vi "Control_Turbi_BIn.vi"(0 "Manual_Off":T1, 1 "Estados_IN":bool[](array[boolean]), 7 "Error In":errorcluster, 8 "T-On (s)":dbl) -> (20 "Estados_OUT":bool[](array[boolean]), 27 "Error Out":errorcluster)   [LabVIEW 2013]
uses:
  Controles/Manual_OFF_TB.ctl
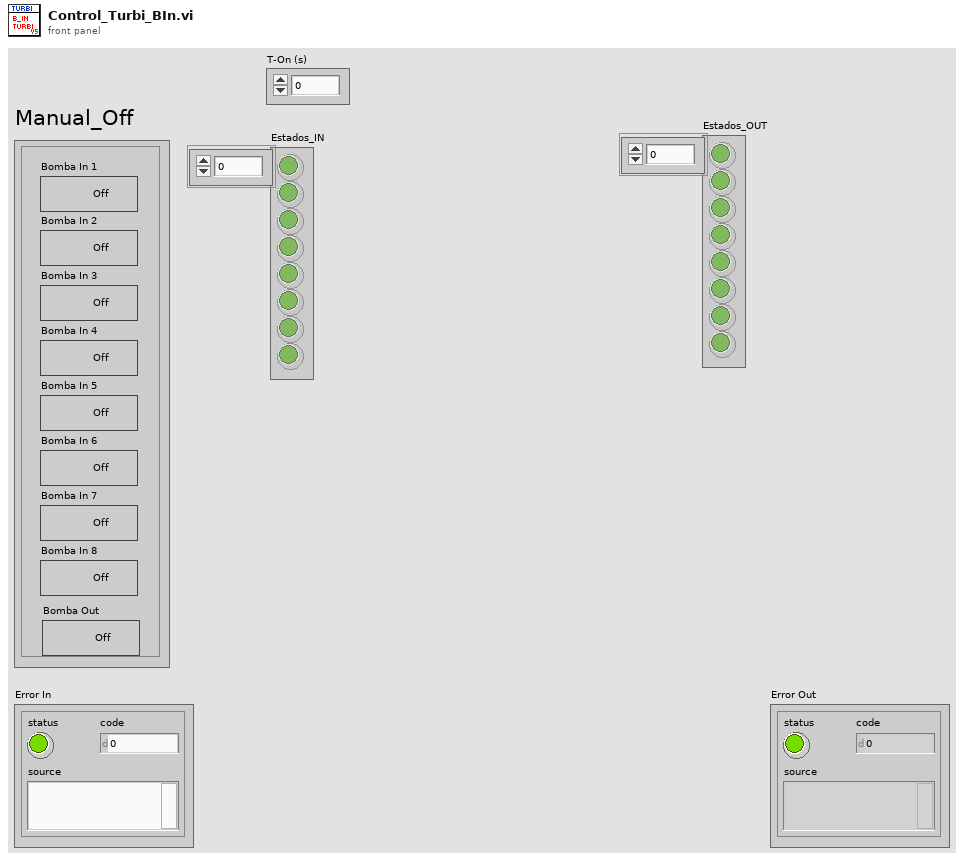
[diagram p1: front panel]
types:
  T1 = typedef "Manual_OFF_TB.ctl" = cluster{"Bomba In 1-1":bool, "Bomba In 1-2":bool, "Bomba In 1-3":bool, "Bomba In 1-4":bool, "Bomba In 1-5":bool, "Bomba In 1-6":bool, "Bomba In 1-7":bool, "Bomba In 1-8":bool, "Bomba Out1":bool}
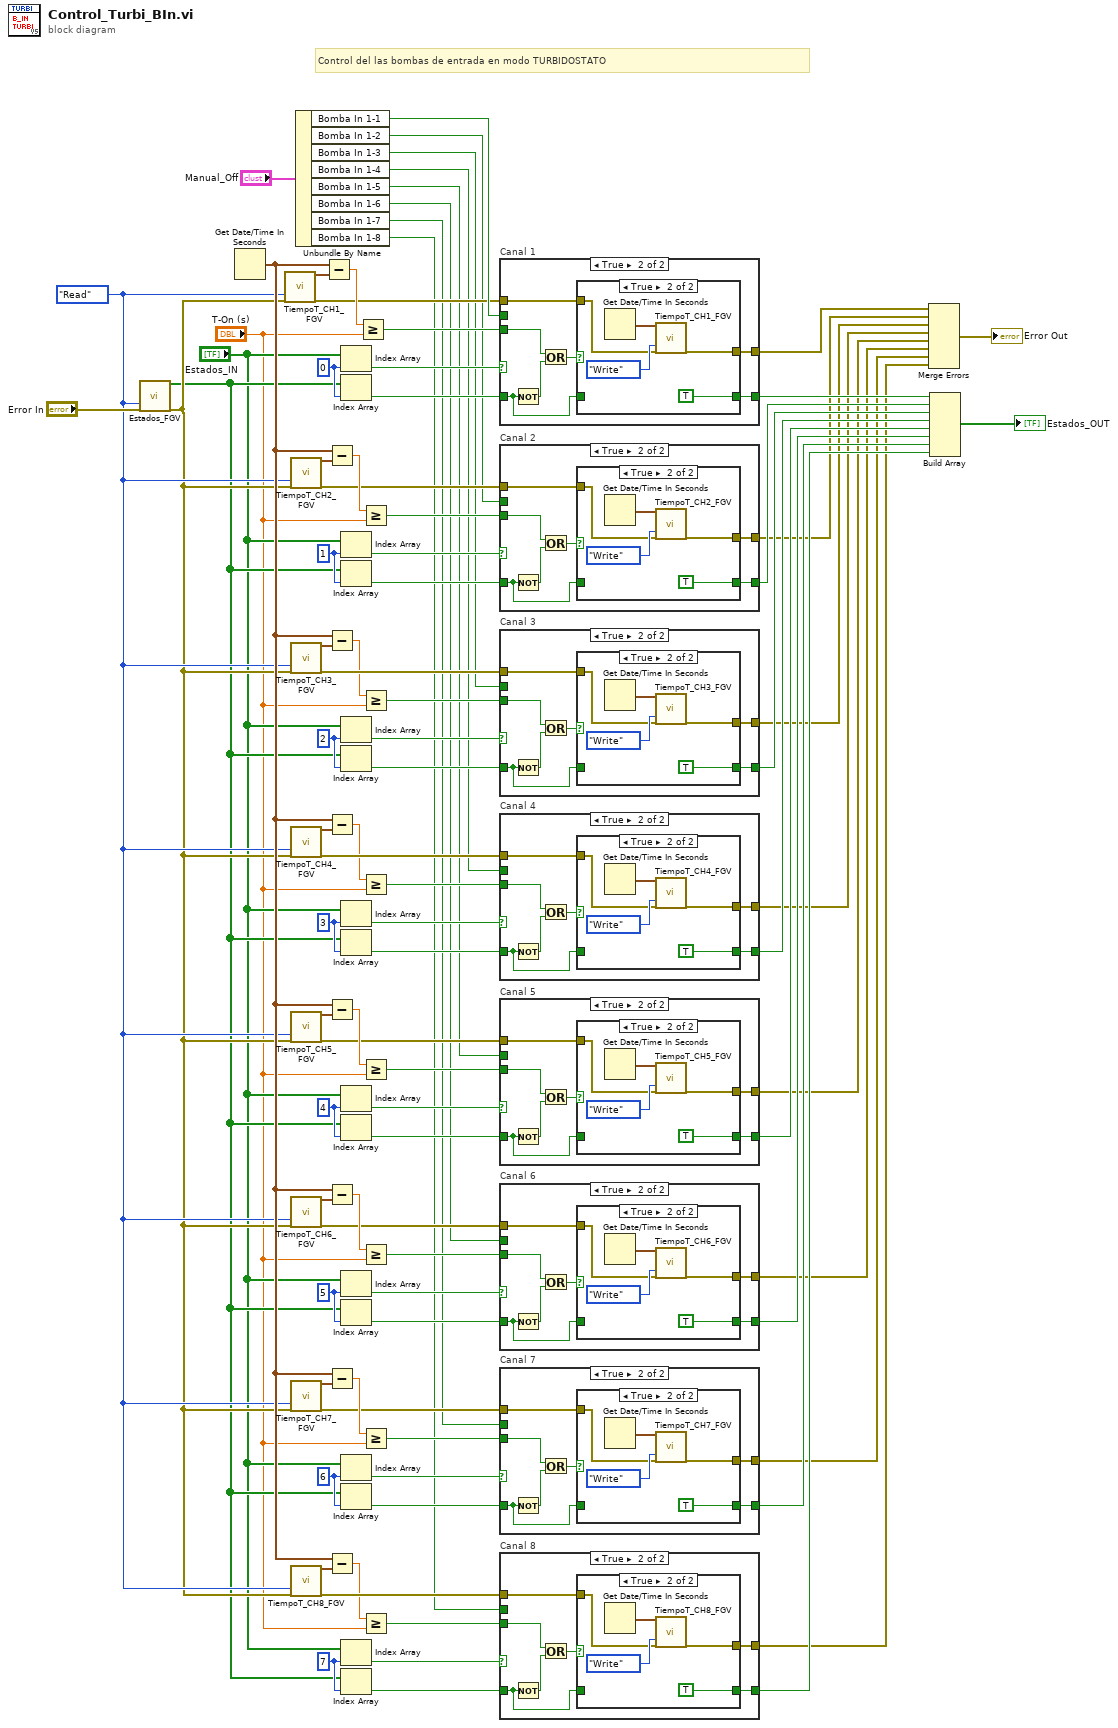
[diagram p0: block diagram]
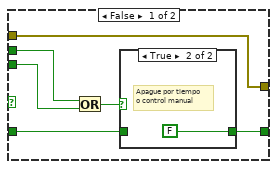
[diagram p2: hidden frame]
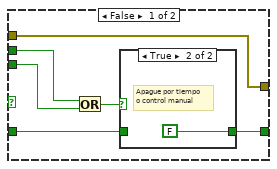
[diagram p5: hidden frame]
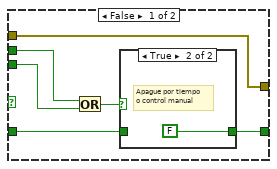
[diagram p8: hidden frame]
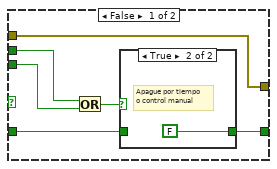
[diagram p11: hidden frame]
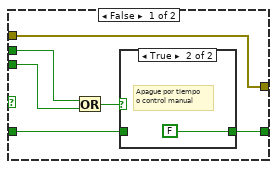
[diagram p14: hidden frame]
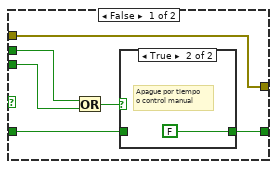
[diagram p17: hidden frame]
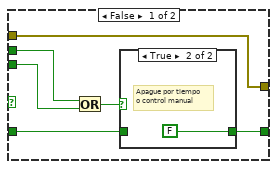
[diagram p20: hidden frame]
diagram:
  w30 = 7 ("index")
  w41 = 6 ("index")
  w27 = 5 ("index")
  w59 = 4 ("index")
  w48 = 3 ("index")
  w64 = 2 ("index")
  w77 = 1 ("index")
  w17 = enum16{"Write", "Read"}."Read" ("Opción")
  w82 = 0 ("index")
  # "Control del las bombas de entrada en modo TURBIDOSTATO"
  n1 = call "Estados_FGV.vi"("Opción"=w17, "Error In"="Error In") -> ("Estados_OUT"=w15:bool[], "Error Out"=w16:errorcluster)  [unwired: 16 in]
  n2 = Get Date/Time In Seconds() -> (seconds since 1Jan1904=w18:timestamp)
  n3 = call "TiempoT_CH1_FGV.vi"("Opción"=w17, "Error In"=w16) -> ("Tiempo_OUT"=w89:timestamp, "Error Out"=w84:errorcluster)  [unwired: 15 in, 1 out]
  n4 = call "TiempoT_CH2_FGV.vi"("Opción"=w17, "Error In"=w16) -> ("Tiempo_OUT"=w72:timestamp, "Error Out"=w73:errorcluster)  [unwired: 15 in, 1 out]
  n5 = call "TiempoT_CH3_FGV.vi"("Opción"=w17, "Error In"=w16) -> ("Tiempo_OUT"=w69:timestamp, "Error Out"=w68:errorcluster)  [unwired: 15 in, 1 out]
  n6 = call "TiempoT_CH4_FGV.vi"("Opción"=w17, "Error In"=w16) -> ("Tiempo_OUT"=w53:timestamp, "Error Out"=w52:errorcluster)  [unwired: 15 in, 1 out]
  n7 = call "TiempoT_CH5_FGV.vi"("Opción"=w17, "Error In"=w16) -> ("Tiempo_OUT"=w54:timestamp, "Error Out"=w55:errorcluster)  [unwired: 15 in, 1 out]
  n8 = call "TiempoT_CH6_FGV.vi"("Opción"=w17, "Error In"=w16) -> ("Tiempo_OUT"=w22:timestamp, "Error Out"=w23:errorcluster)  [unwired: 15 in, 1 out]
  n9 = call "TiempoT_CH7_FGV.vi"("Opción"=w17, "Error In"=w16) -> ("Tiempo_OUT"=w36:timestamp, "Error Out"=w37:errorcluster)  [unwired: 15 in, 1 out]
  n10 = call "TiempoT_CH8_FGV.vi"("Opción"=w17, "Error In"=w16) -> ("Tiempo_OUT"=w35:timestamp, "Error Out"=w34:errorcluster)  [unwired: 15 in, 1 out]
  n11 = Unbundle By Name("Manual_Off") -> ("Bomba In 1-1"=w85:bool, "Bomba In 1-2"=w70:bool, "Bomba In 1-3"=w61:bool, "Bomba In 1-4"=w44:bool, "Bomba In 1-5"=w43:bool, "Bomba In 1-6"=w12:bool, "Bomba In 1-7"=w11:bool, "Bomba In 1-8"=w10:bool)
  n12 = Subtract(x=w18, y=w89) -> (x-y=w88:dbl)
  n13 = Subtract(x=w18, y=w72) -> (x-y=w75:dbl)
  n14 = Subtract(x=w18, y=w69) -> (x-y=w66:dbl)
  n15 = Subtract(x=w18, y=w53) -> (x-y=w50:dbl)
  n16 = Subtract(x=w18, y=w54) -> (x-y=w57:dbl)
  n17 = Subtract(x=w18, y=w22) -> (x-y=w25:dbl)
  n18 = Subtract(x=w18, y=w36) -> (x-y=w39:dbl)
  n19 = Subtract(x=w18, y=w35) -> (x-y=w32:dbl)
  n20 = Index Array(array="Estados_IN", index=w82) -> (element=w90:bool)
  n21 = Index Array(array=w15, index=w82) -> (element=w81:bool)
  n22 = Index Array(array="Estados_IN", index=w77) -> (element=w74:bool)
  n23 = Index Array(array=w15, index=w77) -> (element=w78:bool)
  n24 = Index Array(array="Estados_IN", index=w64) -> (element=w67:bool)
  n25 = Index Array(array=w15, index=w64) -> (element=w63:bool)
  n26 = Index Array(array="Estados_IN", index=w48) -> (element=w51:bool)
  n27 = Index Array(array=w15, index=w48) -> (element=w47:bool)
  n28 = Index Array(array="Estados_IN", index=w59) -> (element=w56:bool)
  n29 = Index Array(array=w15, index=w59) -> (element=w60:bool)
  n30 = Index Array(array="Estados_IN", index=w27) -> (element=w24:bool)
  n31 = Index Array(array=w15, index=w27) -> (element=w28:bool)
  n32 = Index Array(array="Estados_IN", index=w41) -> (element=w38:bool)
  n33 = Index Array(array=w15, index=w41) -> (element=w42:bool)
  n34 = Index Array(array="Estados_IN", index=w30) -> (element=w33:bool)
  n35 = Index Array(array=w15, index=w30) -> (element=w29:bool)
  n36 = Greater Or Equal?(x=w88, y="T-On (s)") -> (x >= y?=w87:bool)
  n37 = Greater Or Equal?(x=w75, y="T-On (s)") -> (x >= y?=w76:bool)
  n38 = Greater Or Equal?(x=w66, y="T-On (s)") -> (x >= y?=w65:bool)
  n39 = Greater Or Equal?(x=w50, y="T-On (s)") -> (x >= y?=w49:bool)
  n40 = Greater Or Equal?(x=w57, y="T-On (s)") -> (x >= y?=w58:bool)
  n41 = Greater Or Equal?(x=w25, y="T-On (s)") -> (x >= y?=w26:bool)
  n42 = Greater Or Equal?(x=w39, y="T-On (s)") -> (x >= y?=w40:bool)
  n43 = Greater Or Equal?(x=w32, y="T-On (s)") -> (x >= y?=w31:bool)
  n44 = case "Canal 1" shown="True" w90 {
    tunnel: w87 -> [w95 w104]
    tunnel: w85 -> [w96 _]
    tunnel: [w93 w101] -> w80
    tunnel: w84 -> [w91 w100]
    tunnel: w81 -> [w92 w102]
    tunnel: [w91 w99] -> w8
    frame False {
      n45 = Or(x=w96, y=w95) -> (x .or. y?=w94:bool)
      n46 = case shown="True" w94 {
        tunnel: [w97 FALSE] -> w93
        tunnel: w92 -> [w97 _]
        frame False {
          # "Mantenga estado"
        }
        frame True {
          # "Apague por tiempo\no control manual"
        }
      }
    }
    frame True {
      n47 = Not(x=w102) -> (.not. x?=w105:bool)
      n48 = Or(x=w104, y=w105) -> (x .or. y?=w103:bool)
      n49 = case shown="True" w103 {
        tunnel: w102 -> [w107 _]
        tunnel: [w107 TRUE ("Boolean")] -> w101
        tunnel: w100 -> [w106 w110]
        tunnel: [w106 w109] -> w99
        frame False {
        }
        frame True {
          n50 = Get Date/Time In Seconds() -> (seconds since 1Jan1904=w108:timestamp)
          n51 = call "TiempoT_CH1_FGV.vi"("Tiempo_IN"=w108, "Opción"=enum16{"Write", "Read"}."Write", "Error In"=w110) -> ("Error Out"=w109:errorcluster)  [unwired: 14 in, 2 out]
        }
      }
    }
  }
  n52 = case "Canal 2" shown="True" w74 {
    tunnel: w76 -> [w117 w126]
    tunnel: w70 -> [w118 _]
    tunnel: [w115 w123] -> w71
    tunnel: w73 -> [w113 w122]
    tunnel: w78 -> [w114 w124]
    tunnel: [w113 w121] -> w7
    frame False {
      n53 = Or(x=w118, y=w117) -> (x .or. y?=w116:bool)
      n54 = case shown="True" w116 {
        tunnel: [w119 FALSE] -> w115
        tunnel: w114 -> [w119 _]
        frame False {
          # "Mantenga estado"
        }
        frame True {
          # "Apague por tiempo\no control manual"
        }
      }
    }
    frame True {
      n55 = Not(x=w124) -> (.not. x?=w127:bool)
      n56 = Or(x=w126, y=w127) -> (x .or. y?=w125:bool)
      n57 = case shown="True" w125 {
        tunnel: w124 -> [w129 _]
        tunnel: [w129 TRUE ("Boolean")] -> w123
        tunnel: w122 -> [w128 w132]
        tunnel: [w128 w131] -> w121
        frame False {
        }
        frame True {
          n58 = Get Date/Time In Seconds() -> (seconds since 1Jan1904=w130:timestamp)
          n59 = call "TiempoT_CH2_FGV.vi"("Tiempo_IN"=w130, "Opción"=enum16{"Write", "Read"}."Write", "Error In"=w132) -> ("Error Out"=w131:errorcluster)  [unwired: 14 in, 2 out]
        }
      }
    }
  }
  n60 = case "Canal 3" shown="True" w67 {
    tunnel: w65 -> [w139 w148]
    tunnel: w61 -> [w140 _]
    tunnel: [w137 w145] -> w62
    tunnel: w68 -> [w135 w144]
    tunnel: w63 -> [w136 w146]
    tunnel: [w135 w143] -> w6
    frame False {
      n61 = Or(x=w140, y=w139) -> (x .or. y?=w138:bool)
      n62 = case shown="True" w138 {
        tunnel: [w141 FALSE] -> w137
        tunnel: w136 -> [w141 _]
        frame False {
          # "Mantenga estado"
        }
        frame True {
          # "Apague por tiempo\no control manual"
        }
      }
    }
    frame True {
      n63 = Not(x=w146) -> (.not. x?=w149:bool)
      n64 = Or(x=w148, y=w149) -> (x .or. y?=w147:bool)
      n65 = case shown="True" w147 {
        tunnel: w146 -> [w151 _]
        tunnel: [w151 TRUE ("Boolean")] -> w145
        tunnel: w144 -> [w150 w154]
        tunnel: [w150 w153] -> w143
        frame False {
        }
        frame True {
          n66 = Get Date/Time In Seconds() -> (seconds since 1Jan1904=w152:timestamp)
          n67 = call "TiempoT_CH3_FGV.vi"("Tiempo_IN"=w152, "Opción"=enum16{"Write", "Read"}."Write", "Error In"=w154) -> ("Error Out"=w153:errorcluster)  [unwired: 14 in, 2 out]
        }
      }
    }
  }
  n68 = case "Canal 4" shown="True" w51 {
    tunnel: w49 -> [w161 w170]
    tunnel: w44 -> [w162 _]
    tunnel: [w159 w167] -> w46
    tunnel: w52 -> [w157 w166]
    tunnel: w47 -> [w158 w168]
    tunnel: [w157 w165] -> w5
    frame False {
      n69 = Or(x=w162, y=w161) -> (x .or. y?=w160:bool)
      n70 = case shown="True" w160 {
        tunnel: [w163 FALSE] -> w159
        tunnel: w158 -> [w163 _]
        frame False {
          # "Mantenga estado"
        }
        frame True {
          # "Apague por tiempo\no control manual"
        }
      }
    }
    frame True {
      n71 = Not(x=w168) -> (.not. x?=w171:bool)
      n72 = Or(x=w170, y=w171) -> (x .or. y?=w169:bool)
      n73 = case shown="True" w169 {
        tunnel: w168 -> [w173 _]
        tunnel: [w173 TRUE ("Boolean")] -> w167
        tunnel: w166 -> [w172 w176]
        tunnel: [w172 w175] -> w165
        frame False {
        }
        frame True {
          n74 = Get Date/Time In Seconds() -> (seconds since 1Jan1904=w174:timestamp)
          n75 = call "TiempoT_CH4_FGV.vi"("Tiempo_IN"=w174, "Opción"=enum16{"Write", "Read"}."Write", "Error In"=w176) -> ("Error Out"=w175:errorcluster)  [unwired: 14 in, 2 out]
        }
      }
    }
  }
  n76 = case "Canal 5" shown="True" w56 {
    tunnel: w58 -> [w183 w192]
    tunnel: w43 -> [w184 _]
    tunnel: [w181 w189] -> w45
    tunnel: w55 -> [w179 w188]
    tunnel: w60 -> [w180 w190]
    tunnel: [w179 w187] -> w4
    frame False {
      n77 = Or(x=w184, y=w183) -> (x .or. y?=w182:bool)
      n78 = case shown="True" w182 {
        tunnel: [w185 FALSE] -> w181
        tunnel: w180 -> [w185 _]
        frame False {
          # "Mantenga estado"
        }
        frame True {
          # "Apague por tiempo\no control manual"
        }
      }
    }
    frame True {
      n79 = Not(x=w190) -> (.not. x?=w193:bool)
      n80 = Or(x=w192, y=w193) -> (x .or. y?=w191:bool)
      n81 = case shown="True" w191 {
        tunnel: w190 -> [w195 _]
        tunnel: [w195 TRUE ("Boolean")] -> w189
        tunnel: w188 -> [w194 w198]
        tunnel: [w194 w197] -> w187
        frame False {
        }
        frame True {
          n82 = Get Date/Time In Seconds() -> (seconds since 1Jan1904=w196:timestamp)
          n83 = call "TiempoT_CH5_FGV.vi"("Tiempo_IN"=w196, "Opción"=enum16{"Write", "Read"}."Write", "Error In"=w198) -> ("Error Out"=w197:errorcluster)  [unwired: 14 in, 2 out]
        }
      }
    }
  }
  n84 = case "Canal 6" shown="True" w24 {
    tunnel: w26 -> [w205 w214]
    tunnel: w12 -> [w206 _]
    tunnel: [w203 w211] -> w21
    tunnel: w23 -> [w201 w210]
    tunnel: w28 -> [w202 w212]
    tunnel: [w201 w209] -> w3
    frame False {
      n85 = Or(x=w206, y=w205) -> (x .or. y?=w204:bool)
      n86 = case shown="True" w204 {
        tunnel: [w207 FALSE] -> w203
        tunnel: w202 -> [w207 _]
        frame False {
          # "Mantenga estado"
        }
        frame True {
          # "Apague por tiempo\no control manual"
        }
      }
    }
    frame True {
      n87 = Not(x=w212) -> (.not. x?=w215:bool)
      n88 = Or(x=w214, y=w215) -> (x .or. y?=w213:bool)
      n89 = case shown="True" w213 {
        tunnel: w212 -> [w217 _]
        tunnel: [w217 TRUE ("Boolean")] -> w211
        tunnel: w210 -> [w216 w220]
        tunnel: [w216 w219] -> w209
        frame False {
        }
        frame True {
          n90 = Get Date/Time In Seconds() -> (seconds since 1Jan1904=w218:timestamp)
          n91 = call "TiempoT_CH6_FGV.vi"("Tiempo_IN"=w218, "Opción"=enum16{"Write", "Read"}."Write", "Error In"=w220) -> ("Error Out"=w219:errorcluster)  [unwired: 14 in, 2 out]
        }
      }
    }
  }
  n92 = case "Canal 7" shown="True" w38 {
    tunnel: w40 -> [w227 w236]
    tunnel: w11 -> [w228 _]
    tunnel: [w225 w233] -> w20
    tunnel: w37 -> [w223 w232]
    tunnel: w42 -> [w224 w234]
    tunnel: [w223 w231] -> w2
    frame False {
      n93 = Or(x=w228, y=w227) -> (x .or. y?=w226:bool)
      n94 = case shown="True" w226 {
        tunnel: [w229 FALSE] -> w225
        tunnel: w224 -> [w229 _]
        frame False {
          # "Mantenga estado"
        }
        frame True {
          # "Apague por tiempo\no control manual"
        }
      }
    }
    frame True {
      n95 = Not(x=w234) -> (.not. x?=w237:bool)
      n96 = Or(x=w236, y=w237) -> (x .or. y?=w235:bool)
      n97 = case shown="True" w235 {
        tunnel: w234 -> [w239 _]
        tunnel: [w239 TRUE ("Boolean")] -> w233
        tunnel: w232 -> [w238 w242]
        tunnel: [w238 w241] -> w231
        frame False {
        }
        frame True {
          n98 = Get Date/Time In Seconds() -> (seconds since 1Jan1904=w240:timestamp)
          n99 = call "TiempoT_CH7_FGV.vi"("Tiempo_IN"=w240, "Opción"=enum16{"Write", "Read"}."Write", "Error In"=w242) -> ("Error Out"=w241:errorcluster)  [unwired: 14 in, 2 out]
        }
      }
    }
  }
  n100 = case "Canal 8" shown="True" w33 {
    tunnel: w31 -> [w249 w258]
    tunnel: w10 -> [w250 _]
    tunnel: [w247 w255] -> w19
    tunnel: w34 -> [w245 w254]
    tunnel: w29 -> [w246 w256]
    tunnel: [w245 w253] -> w1
    frame False {
      n101 = Or(x=w250, y=w249) -> (x .or. y?=w248:bool)
      n102 = case shown="True" w248 {
        tunnel: [w251 FALSE] -> w247
        tunnel: w246 -> [w251 _]
        frame False {
          # "Mantenga estado"
        }
        frame True {
          # "Apague por tiempo\no control manual"
        }
      }
    }
    frame True {
      n103 = Not(x=w256) -> (.not. x?=w259:bool)
      n104 = Or(x=w258, y=w259) -> (x .or. y?=w257:bool)
      n105 = case shown="True" w257 {
        tunnel: w256 -> [w261 _]
        tunnel: [w261 TRUE ("Boolean")] -> w255
        tunnel: w254 -> [w260 w264]
        tunnel: [w260 w263] -> w253
        frame False {
        }
        frame True {
          n106 = Get Date/Time In Seconds() -> (seconds since 1Jan1904=w262:timestamp)
          n107 = call "TiempoT_CH8_FGV.vi"("Tiempo_IN"=w262, "Opción"=enum16{"Write", "Read"}."Write", "Error In"=w264) -> ("Error Out"=w263:errorcluster)  [unwired: 14 in, 2 out]
        }
      }
    }
  }
  n108 = Merge Errors(w8, w7, w6, w5, w4, w3, w2, w1) -> (→"Error Out":errorcluster)
  n109 = Build Array(w80, w71, w62, w46, w45, w21, w20, w19) -> (→"Estados_OUT":bool[])
